vi "Start Command.vi"(8 "error in (no error)":errorcluster, 10 "Robot Actors.lvlib:Command.lvlib:Command.lvclass":refnum<class "Command Actor.lvclass">, 11 "System Actor in":refnum<class "System Actor.lvclass">) -> (0 "error out":errorcluster, 3 "System Actor out":refnum<class "System Actor.lvclass">)   [LabVIEW 2014, in "Robot Actor Framework.lvlib" / "System Actor.lvlib" / "System Actor.lvclass"]
uses:
  System Actor.lvclass
  Command Actor/Command Actor Class/Command Actor.lvclass
  Command Processor Actor/Command Processor Actor Messages/Start Command/Start Command Msg.lvclass/Start Command Msg.ctl
  <vilib>/ActorFramework/Message Enqueuer/Message Enqueuer.lvclass/Message Enqueuer.ctl
  <vilib>/ActorFramework/Message Enqueuer/Enqueue.vi
  <vilib>/ActorFramework/Message Priority Queue/Priority Enqueue.vi
  Command Processor Actor/Command Processor Actor Messages/Start Command/Start Command Msg.lvclass
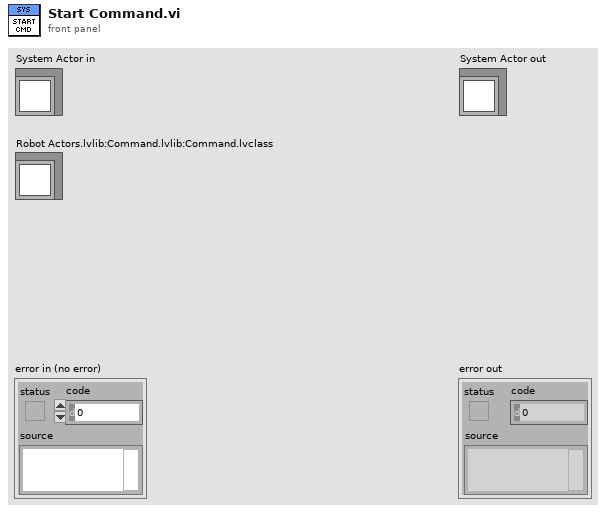
[diagram p1: front panel]
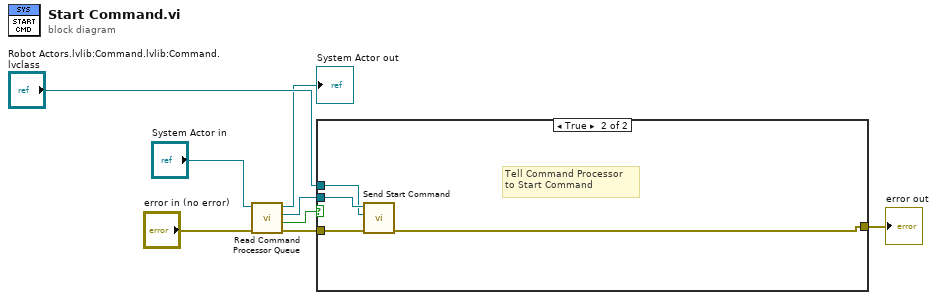
[diagram p0: block diagram]
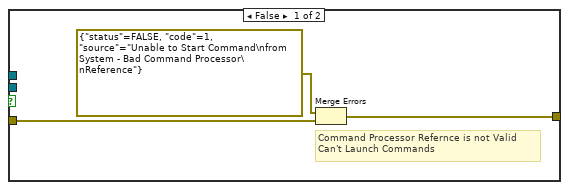
[diagram p2: hidden frame]
diagram:
  n1 = call-dynamic "Read Command Processor Queue.vi"("error in (no error)"="error in (no error)", "System Actor in"="System Actor in") -> ("error out"=w3:errorcluster, "Is Valide Queue?"=w5:bool, "Actor Framework:Message Enqueuer"=w4:refnum<class "Message Enqueuer.lvclass">, "System Actor out"=→"System Actor out":refnum<class "System Actor.lvclass">)  [unwired: 6 in]
  n2 = case shown="True" w5 {
    tunnel: w4 -> [_ w15]
    tunnel: "Robot Actors.lvlib:Command.lvlib:Command.lvclass" -> [_ w14]
    tunnel: w3 -> [w11 w13]
    tunnel: [w10 w12] -> w7
    frame False {
      # "Command Processor Refernce is not Valid\nCan't Launch Commands"
      n3 = Merge Errors(errorcluster {"status"=FALSE, "code"=1, "source"="Unable to Start Command\nfrom System - Bad Command Processor\nReference"} ("error in"), w11) -> (w10:errorcluster)
    }
    frame True {
      # "Tell Command Processor\nto Start Command"
      n4 = call "Send Start Command.vi"("error in (no error)"=w13, "Robot Actors.lvlib:Command.lvlib:Command.lvclass"=w14, "Message Enqueuer"=w15) -> ("error out"=w12:errorcluster)  [unwired: 7 in, 1 out]
    }
  }
  "error out" <- w7
